vi "PathPlanner_PathConstraints_UnlimitedConstraints.vi"(11 "NominalVoltage":dbl=12.0) -> (3 "PathPlannerConstraints":T1)   [LabVIEW 2019, in "PathPlanner24.lvlib"]
doc: "Get unlimited PathConstraints\n\nInputs: \n - NominalVoltageVolts - double - The nominal battery voltage (Volts), default: 12.0\n\n\nOutputs:\n - PathConstraint - cluster - unlimited path constraint data"
uses:
  TypeDef/PathPlannerPathConstraints.ctl
  PathPlanner24.lvlib
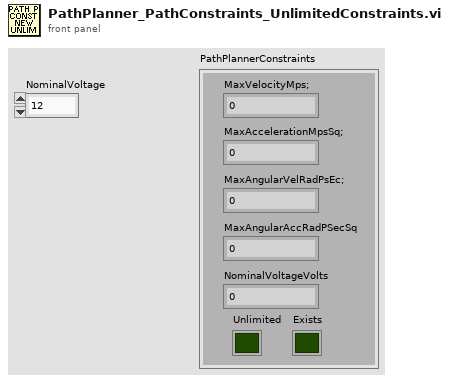
[diagram p1: front panel]
types:
  T1 = typedef "PathPlanner24.lvlib/PathPlannerPathConstraints.ctl" = cluster{"MaxVelocityMps;":dbl, "MaxAccelerationMpsSq;":dbl, "MaxAngularVelRadPsEc;":dbl, "MaxAngularAccRadPSecSq":dbl, "Exists":bool, "Unlimited":bool, "NominalVoltageVolts":dbl}
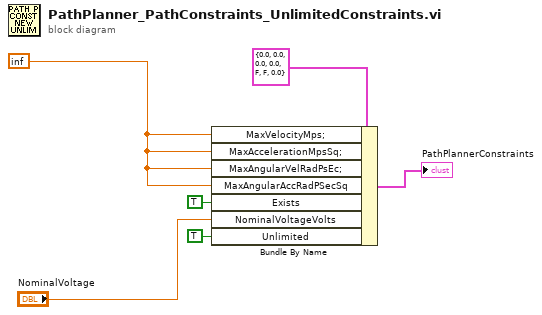
[diagram p0: block diagram]
diagram:
  w2 = inf
  n1 = Bundle By Name(cluster=T1 {"MaxVelocityMps;"=0.0, "MaxAccelerationMpsSq;"=0.0, "MaxAngularVelRadPsEc;"=0.0, "MaxAngularAccRadPSecSq"=0.0, "Exists"=FALSE, "Unlimited"=FALSE, "NominalVoltageVolts"=0.0} ("PathPlannerConstraints"), "MaxVelocityMps;"=w2, "MaxAccelerationMpsSq;"=w2, "MaxAngularVelRadPsEc;"=w2, "MaxAngularAccRadPSecSq"=w2, "Exists"=TRUE, "NominalVoltageVolts"="NominalVoltage", "Unlimited"=TRUE) -> (→"PathPlannerConstraints":T1)
